vi "get Retract wfm.vi"(0 "reference in":refnum<class "Force Curve_tdms.lvclass">, 5 "error in (no error)":errorcluster) -> (14 "reference out":refnum<class "Force Curve_tdms.lvclass">, 16 "Samples retract out":i32, 19 "error out":errorcluster)   [LabVIEW 2019, in "Force Curve_tdms.lvclass"]
uses:
  Force Curve_tdms.lvclass
  private/Signal In.ctl
  <vilib>/Waveform/WDTOps.llb/WDT Get Waveform Subset DBL.vi
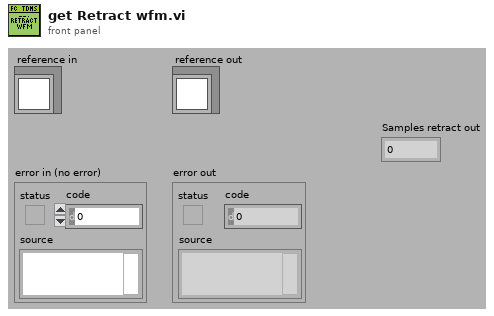
[diagram p1: front panel]
types:
  T1 = typedef "Force Curve_tdms.lvclass/Signal In.ctl" = enum16{"Deflection", "SensorIn", "MockOut", "ZstageOut"}
  T2 = typedef "Force Curve_tdms.lvclass/ObjectAttributesRef.ctl" = refnum<data-value>
  T3 = typedef "Force Curve_tdms.lvclass/ObjectAttributes.ctl" = cluster{"MyAttribute":dbl, "Processed data":waveform(dbl)[], "Fcurve Raw Metadata":T4, "Fcurve Metadata":T5, "Fcurve index":T6, "Tau Delay (ms)":dbl, "Contact Spread of dev":dbl, "Fcurve":T7}
  T4 = typedef "TDMS_DataHandler.lvclass/Fcurve Meta data.ctl" = cluster{"property names":string[], "property values":variant[]}
  T5 = typedef "Force Curve_tdms.lvclass/Fcurve Meta data analysis.ctl" = cluster{"dt (us)":dbl, "Dec Factor":dbl, "Z piezo Sensitivity (nm/V)":dbl, "K (N/m)":dbl, "Sp (V)":dbl, "Contact (ms)":dbl, "Zpos contact":dbl, "Vel_app (nm/s)":dbl, "Vel_ret (nm/s)":dbl, "deltaV (nm)":dbl, "Def_V0 (v)":dbl, "Decimating Factor":dbl}
  T6 = typedef "Force Curve_tdms.lvclass/Fcurve Index .ctl" = cluster{"Setpoint index":i32, "Max force index":i32, "Contact point index":i32, "Appoach indices":cluster{"Start":i32, "End":i32}, "Contact indices":cluster{"Start":i32, "End":i32}, "Retract indices":cluster{"Start":i32, "End":i32}}
  T7 = typedef "Force Curve_tdms.lvclass/Force Curve data.ctl" = cluster{"Approach":cluster{"X":dbl[], "Y":dbl[]}, "Contact":cluster{"X":dbl[], "Y":dbl[]}, "Retract":cluster{"X":dbl[], "Y":dbl[]}}
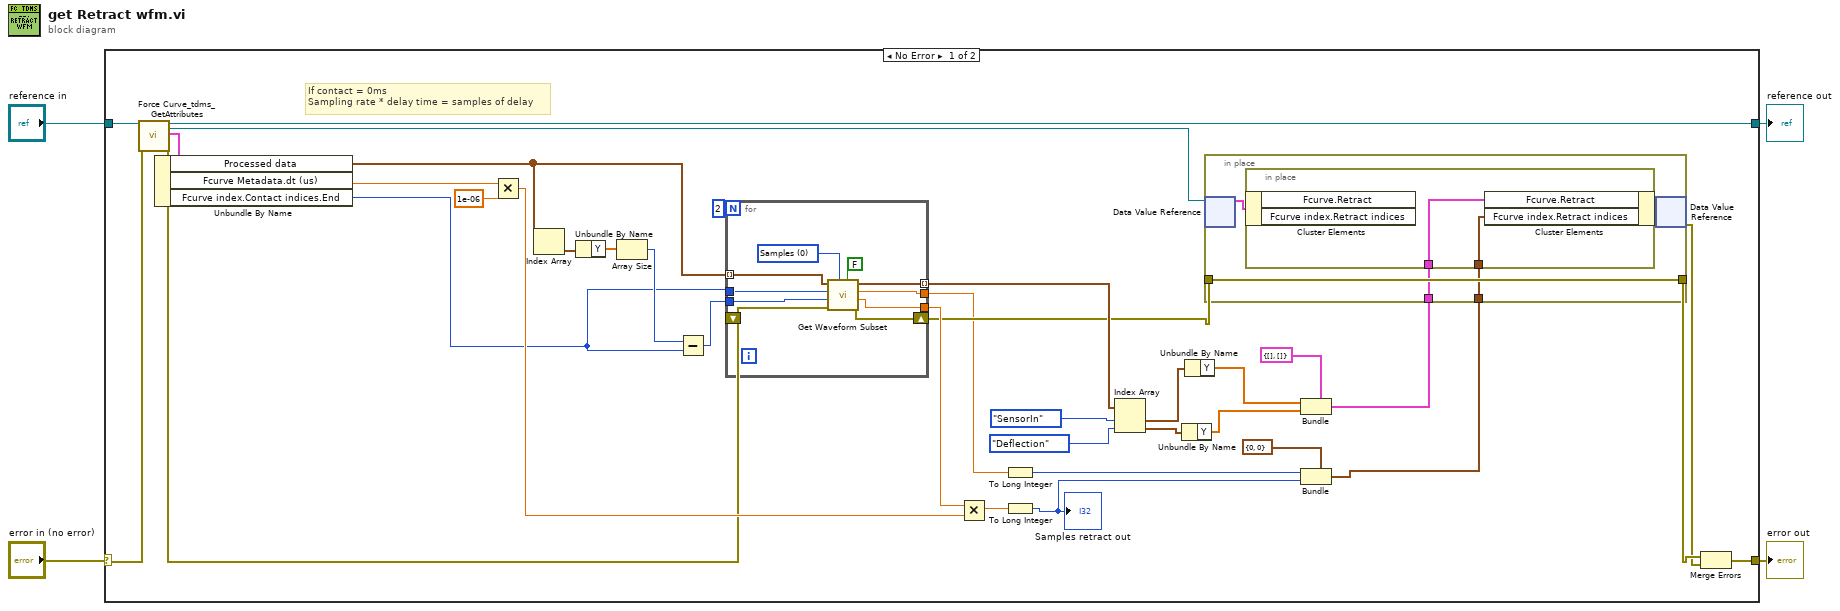
[diagram p0: block diagram]
diagram:
  n1 = case shown="No Error" "error in (no error)" {
    selector: "error in (no error)" -> [w38 w59]
    tunnel: [w40 w59] -> w3
    tunnel: [w39 w58] -> w1
    tunnel: "reference in" -> [w32 w58]
    frame No Error {
      # "If contact = 0ms\nSampling rate * delay time = samples of delay"
      n2 = call "Force Curve_tdms_GetAttributes.vi"("reference in"=w32, "error in (no error)"=w38) -> ("reference out"=w39:refnum<class "Force Curve_tdms.lvclass">, "attributes ref"=w34:T2, "attributes"=w37:T3, "error out"=w10:errorcluster)  [unwired: 14 in]
      n3 = Unbundle By Name(w37) -> ("Processed data"=w18:waveform(dbl)[], "Fcurve Metadata.dt (us)"=w22:dbl, "Fcurve index.Contact indices.End"=w11:i32)
      n4 = Multiply(x=w22, y=1e-06) -> (x*y=w14:dbl)
      n5 = Index Array(array=w18) -> (element=w17:waveform(dbl))  [unwired: 1 in]
      n6 = Unbundle By Name(w17) -> ("Y"=w16:dbl[])
      n7 = Array Size(array=w16) -> (size(s)=w15:i32)
      n8 = Subtract(x=w15, y=w11) -> (x-y=w13:i32)
      n9 = for {
        N: 2 -> [_]
        tunnel: [w49] -> w33
        tunnel: [w48] -> w29 mode=indexing
        tunnel: w18 -> [w47] mode=indexing
        tunnel: w11 -> [w46]
        tunnel: w13 -> [w45]
        shift-right: [w42] -> w12
        shift-left: w10 -> [w43]
        tunnel: [w41] -> w6
        w50 = u16 0 items=["Samples", "Relative Time"] ("start/duration format")
        n10 = call-poly <vilib>:"Get Waveform Subset.vi"("open interval? (T)"=FALSE, "start/duration format"=w50, "error in (no error)"=w43, "duration"=w45, "start samples/time"=w46, "waveform in"=w47) -> ("error out"=w42:errorcluster, "actual duration"=w49:dbl, "actual start samples/time"=w41:dbl, "waveform out"=w48:waveform(dbl))
      }
      n11 = Multiply(x=w33, y=w14) -> (x*y=w19:dbl)
      n12 = To Long Integer(number=w6) -> (32bit integer=w5:i32)
      n13 = To Long Integer(number=w19) -> (32bit integer=w7:i32)
      "Samples retract out" <- w7
      n14 = Index Array(array=w29, index #1=Signal_In."SensorIn" ("Signal in"), index #2=Signal_In."Deflection" ("Signal in")) -> (element #1=w26:waveform(dbl), element #2=w25:waveform(dbl))
      n15 = Unbundle By Name(w25) -> ("Y"=w24:dbl[])
      n16 = Unbundle By Name(w26) -> ("Y"=w23:dbl[])
      n17 = Bundle(cluster=cluster{"X":dbl[], "Y":dbl[]} {"X"=[], "Y"=[]} ("Fcurve.Approach"), "X"=w23, "Y"=w24) -> (w30:cluster{"X":dbl[], "Y":dbl[]})
      n18 = Bundle(cluster=cluster{"Start":i32, "End":i32} {"Start"=0, "End"=0} ("Fcurve index.Retract indices"), "Start"=w5, "End"=w7) -> (w8:cluster{"Start":i32, "End":i32})
      n19 = in-place {
        in-place-border: w12 -> [w53]
        in-place-border: [w53] -> w36
        in-place-border: w30 -> [w52]
        in-place-border: w8 -> [w51]
        n20 = in-place-dvr #1(w34) -> (w54:T3)  [unwired: 1 out]
        n21 = in-place {
          in-place-border: w52 -> [w57]
          in-place-border: w51 -> [w56]
          n22 = in-place-cluster #2(w54) -> ()  [unwired: 2 out]
          n23 = in-place-cluster #2("Fcurve.Retract"=w57, "Fcurve index.Retract indices"=w56) -> (w55:T3)
        }
        n24 = in-place-dvr #1(w55) -> (w35:errorcluster)  [unwired: 1 out]
      }
      n25 = Merge Errors(w36, w35) -> (w40:errorcluster)
    }
    frame Error {
    }
  }
  "error out" <- w3
  "reference out" <- w1
